vi "fpga_Ref Filter (M Class_50Hz).vi"(7 "reset":bool, 9 "input valid":bool, 10 "Memory In":refnum<k21>="coefROM", 11 "input data":fxp<+/-,24,1>) -> (0 "error":i32, 1 "output valid":bool, 3 "output data <i24,3>":fxp<+/-,24,3> format="%.22g", 4 "ready for input":bool)   [LabVIEW 2013, in "NI_EP_PMU_FPGA.lvlib"]
uses:
  <vilib>/addons/Electrical Power/PMU/NI_EP_PMU_FPGA.lvlib
  <vilib>/addons/Electrical Power/PQ/Resampling/NI_EP_Resample_FPGA.lvlib
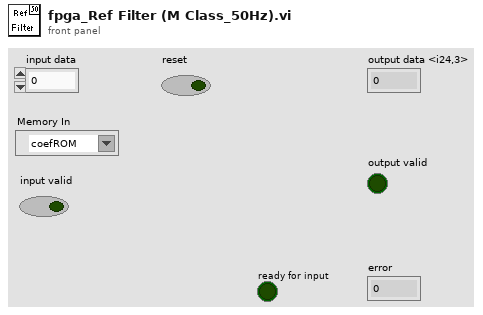
[diagram p1: front panel]
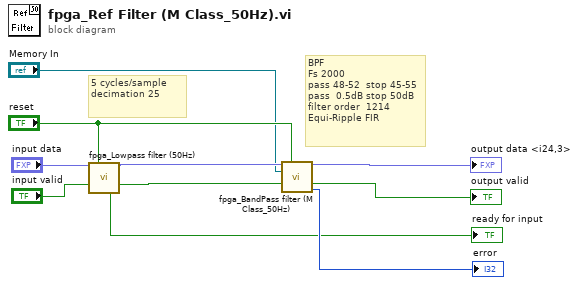
[diagram p0: block diagram]
diagram:
  # "BPF\nFs 2000\npass 48-52  stop 45-55\npass  0.5dB stop 50dB\nfilter order  1214\nEqui-Ripple FIR"
  # "5 cycles/sample\ndecimation 25"
  n1 = call <vilib>:"fpga_Lowpass filter (50Hz).vi"("input data"="input data", "reset"="reset", "input valid"="input valid") -> ("output data"=w8:fxp<+/-,24,2>, "output valid"=w6:bool, "ready for input"=→"ready for input":bool)  [unwired: 10 in]
  n2 = call <vilib>:"fpga_BandPass filter (M Class_50Hz).vi"("input data"=w8, "reset"="reset", "Memory In"="Memory In", "input valid"=w6) -> ("output data"=→"output data <i24,3>":fxp<+/-,24,3>, "output valid"=→"output valid":bool, "error"=→"error":i32)  [unwired: 8 in, 1 out]
